vi "run.vi"(8 "error in (no error)":errorcluster, 11 "Filter_Wheel in":refnum<class "Filter_Wheel.lvclass">) -> (0 "error out":errorcluster, 3 "Filter_Wheel out":refnum<class "Filter_Wheel.lvclass">)   [LabVIEW 2018, in "Filter_Wheel.lvclass"]
uses:
  Filter_Wheel.lvclass
  Filter_Wheel.lvclass/Filter_Wheel.ctl
  State Machine/State Machine.lvclass
  RxTx/RxTx.lvclass
panel:
  out "Select Filter":u16(ring) items=["Methane", "U", "B", "V", "R", "I", "Clear"]
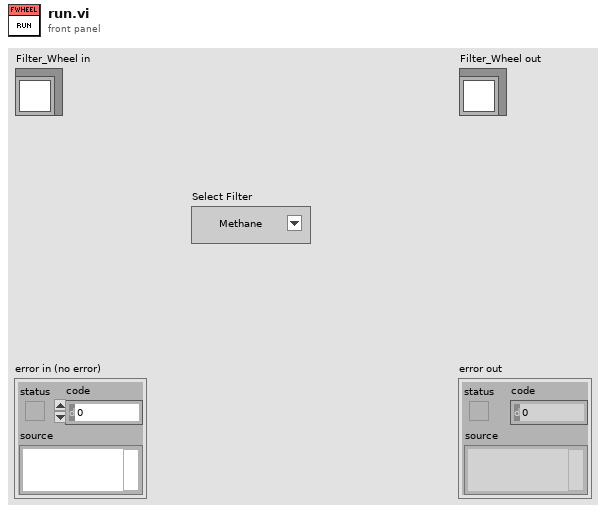
[diagram p1: front panel]
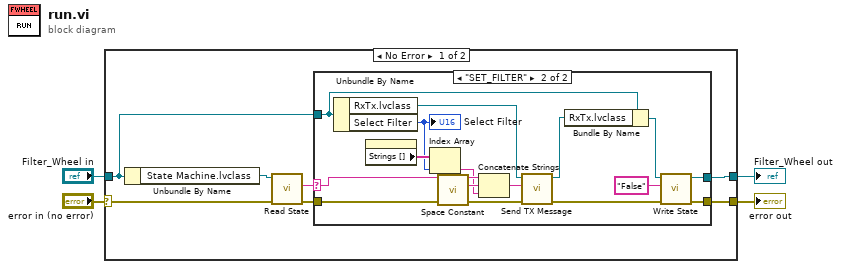
[diagram p0: block diagram]
diagram:
  n1 = case shown="No Error" "error in (no error)" {
    selector: "error in (no error)" -> [w10 w30]
    tunnel: [w5 w30] -> w3
    tunnel: [w6 w29] -> w1
    tunnel: "Filter_Wheel in" -> [w8 w29]
    frame No Error {
      n2 = Unbundle By Name(w8) -> ("State Machine.lvclass"=w11:refnum<class "State Machine.lvclass">)
      n3 = call-dynamic "Read State.vi"("error in (no error)"=w10, "State Machine in"=w11) -> ("error out"=w7:errorcluster, "State"=w9:string)  [unwired: 7 in, 1 out]
      n4 = case shown="\"SET_FILTER\"" w9 {
        selector: w9 -> [_ w27]
        tunnel: w8 -> [w13 w24]
        tunnel: w7 -> [w12 w25]
        tunnel: [w13 w18] -> w6
        tunnel: [w12 w19] -> w5
        frame "False", Default {
        }
        frame "SET_FILTER" {
          n5 = Unbundle By Name(w24) -> ("RxTx.lvclass"=w22:refnum<class "RxTx.lvclass">, "Select Filter"=w15:u16)
          "Select Filter" <- w15
          n6 = property on="Select Filter" class="Ring (strict)"() -> ("Strings []"=w16:string[])  [unwired: 2 in, 2 out]
          n7 = Index Array(array=w16, index=w15) -> (element=w14:string)
          n8 = call <vilib>:"Space Constant.vi"() -> ("String"=w26:string)
          n9 = Concatenate Strings(w27, w26, w14) -> (w28:string)
          n10 = call "Send TX Message.vi"("error in (no error)"=w25, "element"=w28, "RxTx in"=w22) -> ("error out"=w20:errorcluster, "RxTx out"=w23:refnum<class "RxTx.lvclass">)  [unwired: 7 in]
          n11 = Bundle By Name(cluster=w24, "RxTx.lvclass"=w23) -> (w21:refnum<class "Filter_Wheel.lvclass">)
          n12 = call "Write State.vi"("error in (no error)"=w20, "State"="False", "Filter_Wheel in"=w21) -> ("error out"=w19:errorcluster, "Filter_Wheel out"=w18:refnum<class "Filter_Wheel.lvclass">)  [unwired: 7 in]
        }
      }
    }
    frame Error {
    }
  }
  "error out" <- w3
  "Filter_Wheel out" <- w1
